vi "Color Check.vi"(1 "Color in":u32) -> (0 "Color out":u32)   [LabVIEW 2017, in "Measurement.PhotocurrentMapping.UI.lvclass"]
uses:
  Measurement.PhotocurrentMapping.UI.lvclass
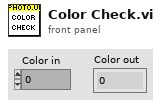
[diagram p1: front panel]
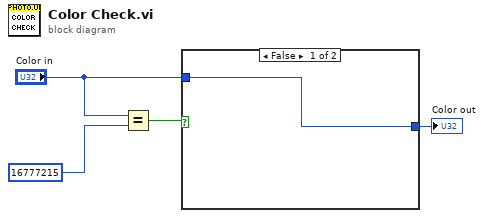
[diagram p0: block diagram]
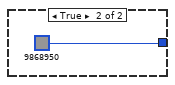
[diagram p2: hidden frame]
diagram:
  n1 = Equal?(x="Color in", y=u32 16777215) -> (x = y?=w3:bool)
  n2 = case shown="False" w3 {
    tunnel: "Color in" -> [w5 _]
    tunnel: [w5 u32 9868950] -> w1
    frame False {
    }
    frame True {
    }
  }
  "Color out" <- w1
